vi "ReadVNAExcel.vi"() -> ()   [LabVIEW 2020]
uses:
  <vilib>/addons/_office/excel.llb/Excel Get Data ([dbl]).vi
  <vilib>/Utility/NIReport.llb/NI_report.lvclass
  <vilib>/Utility/NIReport.llb/Excel/NI_Excel.lvclass
  <vilib>/addons/_office/NI_ReportGenerationToolkit.lvlib
panel:
  out "output cluster":T1
  in  "file path (dialog if empty)":path=path "C:/projects/UNI/VNA/Jorgmalinger20240615/vann0.01M-20240625-505.xlsx"
  out "Output":dbl[][](array[numeric])
  out "Sheet 1 Data":dbl[][](array[numeric]) format="%.2f"
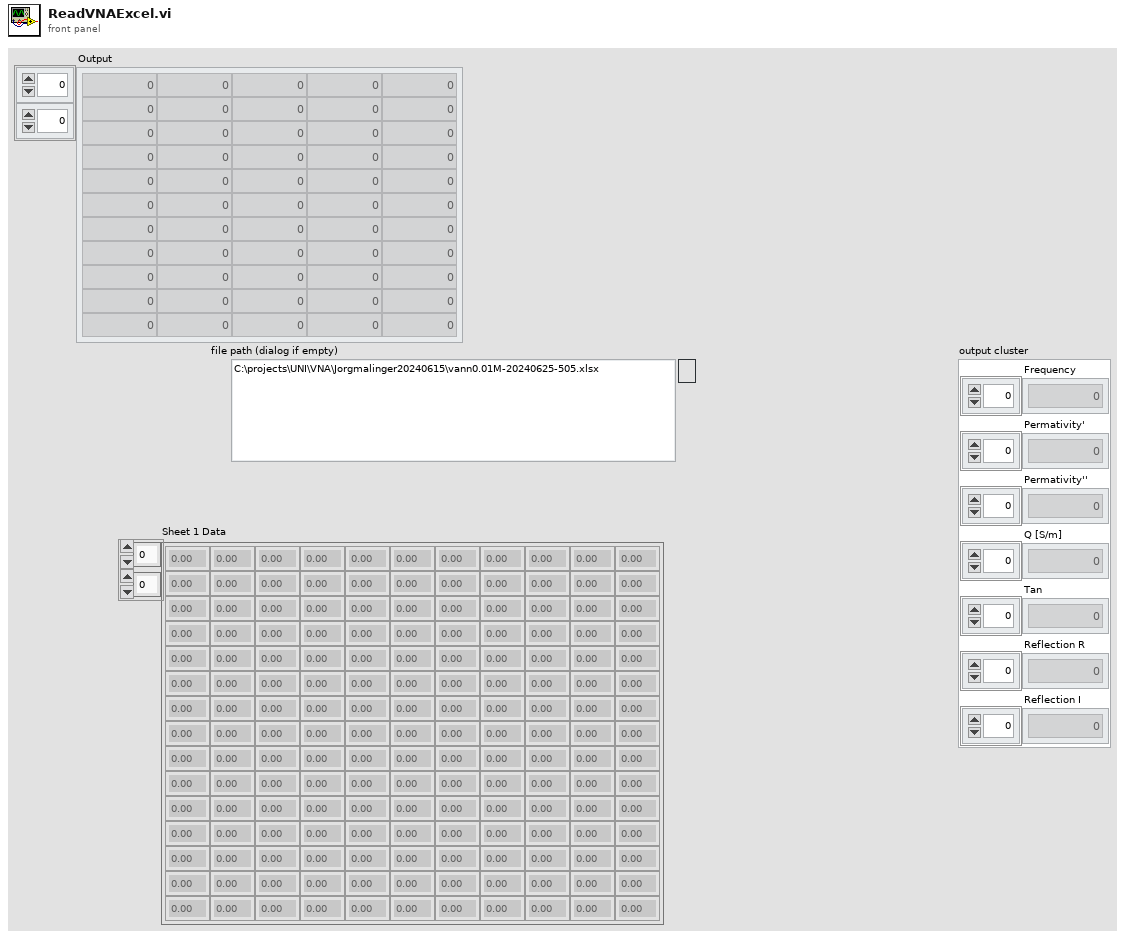
[diagram p1: front panel]
types:
  T1 = cluster{"Frequency":dbl[], "Permativity'":dbl[], "Permativity''":dbl[], "Q [S/m]":dbl[], "Tan":dbl[], "Reflection R":dbl[], "Reflection I":dbl[]}
  T2 = enum16{"Standard Report", "HTML", "Word", "Excel"}
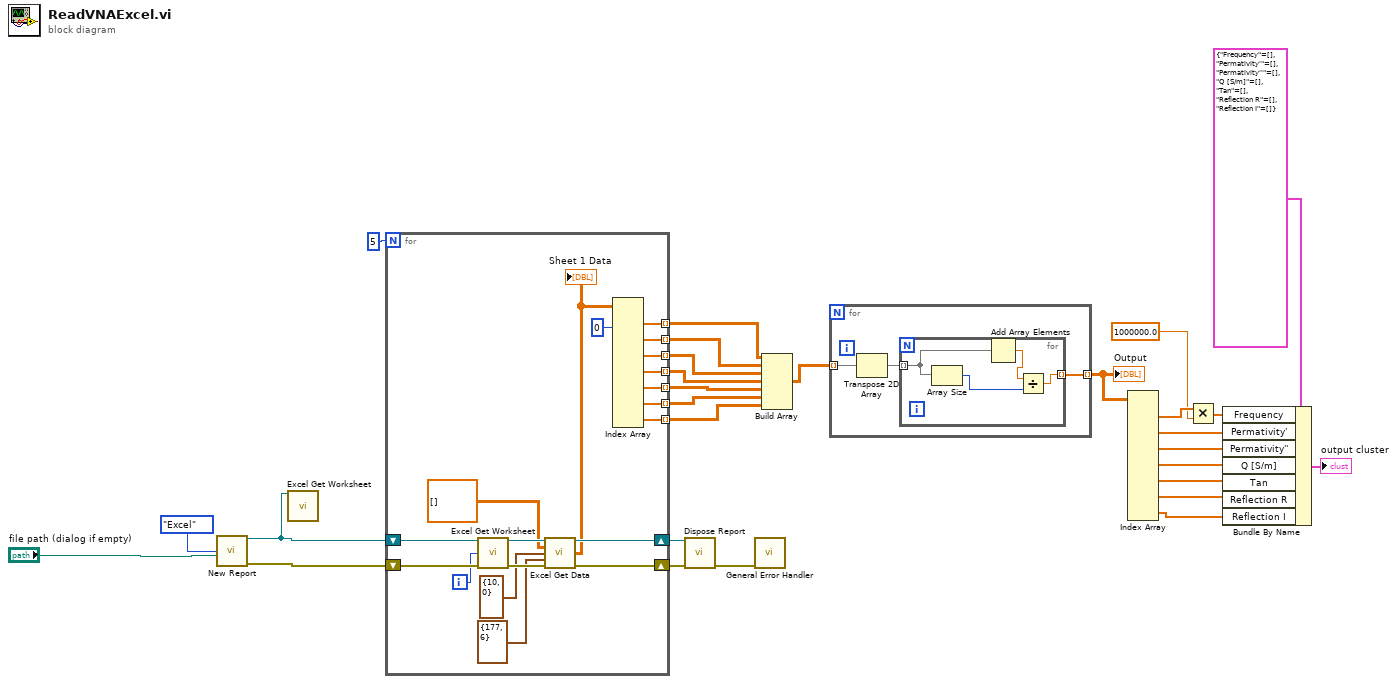
[diagram p0: block diagram]
diagram:
  n1 = call <vilib>:"New Report.vi"("report type"=T2."Excel", "template (empty)"="file path (dialog if empty)") -> ("report out"=w1:refnum<class "NI_report.lvclass">, "error out"=w26:errorcluster)  [unwired: 4 in, 8 out]
  n2 = call <vilib>:"Excel Get Worksheet.vi"("report in"=w1) -> ()  [unwired: 2 in, 13 out]
  n3 = for {
    N: 5 -> [_]
    shift-right: [w44] -> w27
    shift-left: w1 -> [w47]
    shift-right: [w40] -> w24
    shift-left: w26 -> [w43]
    tunnel: [w37] -> w21 mode=indexing
    tunnel: [w34] -> w20 mode=indexing
    tunnel: [w33] -> w18 mode=indexing
    tunnel: [w32] -> w17 mode=indexing
    tunnel: [w31] -> w16 mode=indexing
    tunnel: [w30] -> w15 mode=indexing
    tunnel: [w29] -> w14 mode=indexing
    i -> [w38]
    n4 = call <vilib>:"Excel Get Worksheet.vi"("report in"=w47, "worksheet index (0)"=w38, "error in (no error)"=w43) -> ("report out"=w46:refnum<class "NI_report.lvclass">, "error out"=w42:errorcluster)  [unwired: 11 out]
    n5 = call-poly <vilib>:"Excel Get Data.vi"("report in"=w46, "data type"=dbl[][] [], "start (-1, -1)"=cluster{"row":i32, "column":i32} {"row"=10, "column"=0}, "end (-1, -1)"=cluster{"row":i32, "column":i32} {"row"=177, "column"=6}, "error in (no error)"=w42) -> ("report out"=w44:refnum<class "NI_report.lvclass">, "data"=w35:dbl[][], "error out"=w40:errorcluster)  [unwired: 8 out]
    "Sheet 1 Data" <- w35
    n6 = Index Array(array=w35, index (col) #1=0 ("disabled index (col)")) -> (element #1=w37:dbl[], element #2=w34:dbl[], element #3=w33:dbl[], element #4=w32:dbl[], element #5=w31:dbl[], element #6=w30:dbl[], element #7=w29:dbl[])  [unwired: 13 in]
  }
  n7 = call-dynamic "Dispose Report.vi"("report in"=w27, "error in (no error)"=w24) -> ("error out"=w25:errorcluster)  [unwired: 3 in, 10 out]
  n8 = call <vilib>:"General Error Handler.vi"("error in (no error)"=w25) -> ()  [unwired: 3 in, 12 out]
  n9 = Build Array(w21, w20, w18, w17, w16, w15, w14) -> (w19:dbl[][][])
  n10 = for {
    tunnel: w19 -> [w48] mode=indexing
    tunnel: [w49] -> w13 mode=indexing
    n11 = Transpose 2D Array(2D array=w48) -> (transposed array=w50:dbl[][])
    n12 = for {
      tunnel: w50 -> [w54] mode=indexing
      tunnel: [w53] -> w49 mode=indexing
      n13 = Array Size(array=w54) -> (size(s)=w51:i32)
      n14 = Add Array Elements(numeric array=w54) -> (sum=w52:dbl)
      n15 = Divide(x=w52, y=w51) -> (x/y=w53:dbl)
    }
  }
  "Output" <- w13
  n16 = Index Array(array=w13) -> (element #1=w11:dbl[], element #2=w10:dbl[], element #3=w9:dbl[], element #4=w8:dbl[], element #5=w7:dbl[], element #6=w6:dbl[], element #7=w5:dbl[])  [unwired: 14 in]
  n17 = Multiply(x=w11, y=1000000.0) -> (x*y=w3:dbl[])
  n18 = Bundle By Name(cluster=T1 {"Frequency"=[], "Permativity'"=[], "Permativity''"=[], "Q [S/m]"=[], "Tan"=[], "Reflection R"=[], "Reflection I"=[]}, "Frequency"=w3, "Permativity'"=w10, "Permativity''"=w9, "Q [S/m]"=w8, "Tan"=w7, "Reflection R"=w6, "Reflection I"=w5) -> (→"output cluster":T1)
